vi "PrepSweepCurr.vi"(4 "OC protection":bool, 5 "Voltage/Current Limit (0V/A)":dbl, 6 "OV protection":bool, 7 "OV Value (10V)":dbl=10.0, 8 "error in (no error)":errorcluster, 9 "CC (1)/VC (0)":bool, 10 "Start Current/Voltage (0 A/V)":dbl, 11 "VISA resource name":refnum<visa-resource-name>) -> (0 "error out":errorcluster, 3 "VISA resource name out":refnum<visa-resource-name>)   [LabVIEW 2017]
doc: "Configures the current transient mode and output current level."
uses:
  Keysight N8731A conversion/Keysight N8900 Series.lvlib
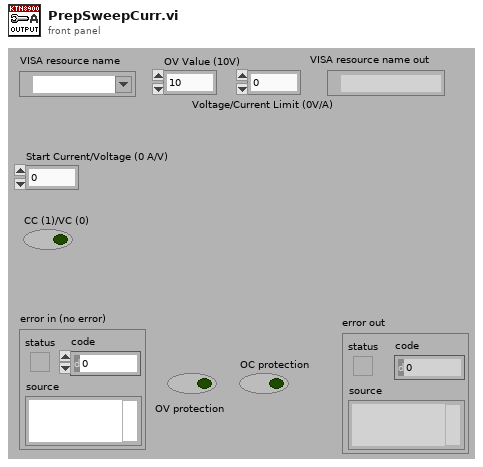
[diagram p1: front panel]
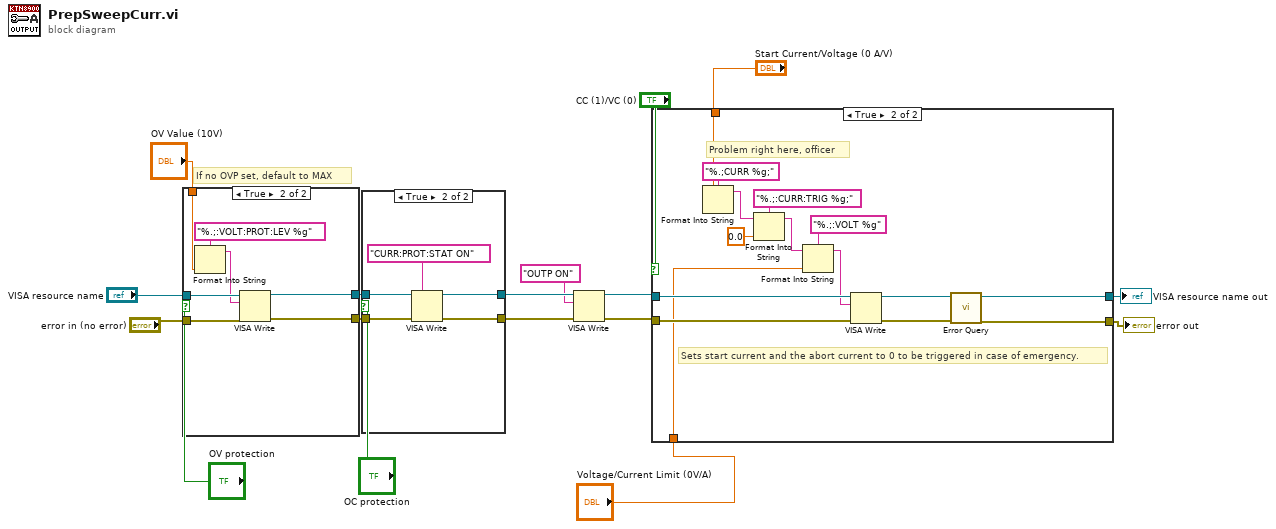
[diagram p0: block diagram]
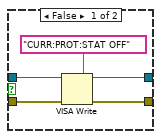
[diagram p2: hidden frame]
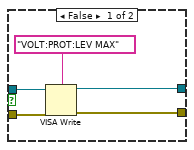
[diagram p3: hidden frame]
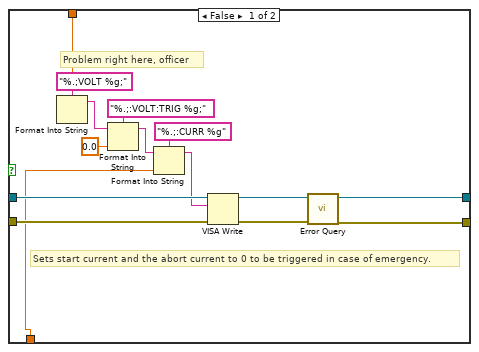
[diagram p4: hidden frame]
diagram:
  # "If no OVP set, default to MAX"
  n1 = case shown="True" "OV protection" {
    tunnel: "VISA resource name" -> [w22 w29]
    tunnel: "error in (no error)" -> [w21 w28]
    tunnel: [w19 w27] -> w13
    tunnel: [w20 w26] -> w12
    tunnel: "OV Value (10V)" -> [_ w23]
    frame False {
      n2 = VISA Write(VISA resource name=w22, write buffer="VOLT:PROT:LEV MAX", error in (no error)=w21) -> (VISA resource name out=w19:refnum<visa-resource-name>, error out=w20:errorcluster)  [unwired: 1 out]
    }
    frame True {
      n3 = Format Into String(format string="%.;:VOLT:PROT:LEV %g", w23) -> (resulting string=w24:string)  [unwired: 2 in, 1 out]
      n4 = VISA Write(VISA resource name=w29, write buffer=w24, error in (no error)=w28) -> (VISA resource name out=w27:refnum<visa-resource-name>, error out=w26:errorcluster)  [unwired: 1 out]
    }
  }
  n5 = case shown="True" "OC protection" {
    tunnel: w13 -> [w33 w39]
    tunnel: w12 -> [w32 w38]
    tunnel: [w31 w37] -> w5
    tunnel: [w30 w36] -> w4
    frame False {
      n6 = VISA Write(VISA resource name=w33, write buffer="CURR:PROT:STAT OFF", error in (no error)=w32) -> (VISA resource name out=w31:refnum<visa-resource-name>, error out=w30:errorcluster)  [unwired: 1 out]
    }
    frame True {
      n7 = VISA Write(VISA resource name=w39, write buffer="CURR:PROT:STAT ON", error in (no error)=w38) -> (VISA resource name out=w37:refnum<visa-resource-name>, error out=w36:errorcluster)  [unwired: 1 out]
    }
  }
  n8 = VISA Write(VISA resource name=w5, write buffer="OUTP ON", error in (no error)=w4) -> (VISA resource name out=w3:refnum<visa-resource-name>, error out=w2:errorcluster)  [unwired: 1 out]
  n9 = case shown="True" "CC (1)/VC (0)" {
    tunnel: w3 -> [w54 w69]
    tunnel: w2 -> [w53 w68]
    tunnel: [w50 w65] -> w9
    tunnel: [w49 w64] -> w8
    tunnel: "Start Current/Voltage (0 A/V)" -> [w44 w59]
    tunnel: "Voltage/Current Limit (0V/A)" -> [w42 w57]
    frame False {
      # "Problem right here, officer"
      # "Sets start current and the abort current to 0 to be triggered in case of emergency."
      n10 = Format Into String(format string="%.;VOLT %g;", w44) -> (resulting string=w46:string)  [unwired: 2 in, 1 out]
      n11 = Format Into String(format string="%.;:VOLT:TRIG %g;", initial string=w46, 0.0 ("input 1")) -> (resulting string=w43:string)  [unwired: 1 in, 1 out]
      n12 = Format Into String(format string="%.;:CURR %g", initial string=w43, w42) -> (resulting string=w40:string)  [unwired: 1 in, 1 out]
      n13 = VISA Write(VISA resource name=w54, write buffer=w40, error in (no error)=w53) -> (VISA resource name out=w52:refnum<visa-resource-name>, error out=w51:errorcluster)  [unwired: 1 out]
      n14 = call "Error Query.vi"("error in (no error)"=w51, "VISA resource name"=w52) -> ("error out"=w49:errorcluster, "VISA resource name out"=w50:refnum<visa-resource-name>)  [unwired: 6 in, 2 out]
    }
    frame True {
      # "Problem right here, officer"
      # "Sets start current and the abort current to 0 to be triggered in case of emergency."
      n15 = Format Into String(format string="%.;CURR %g;", w59) -> (resulting string=w61:string)  [unwired: 2 in, 1 out]
      n16 = Format Into String(format string="%.;:CURR:TRIG %g;", initial string=w61, 0.0 ("input 1")) -> (resulting string=w58:string)  [unwired: 1 in, 1 out]
      n17 = Format Into String(format string="%.;:VOLT %g", initial string=w58, w57) -> (resulting string=w56:string)  [unwired: 1 in, 1 out]
      n18 = VISA Write(VISA resource name=w69, write buffer=w56, error in (no error)=w68) -> (VISA resource name out=w67:refnum<visa-resource-name>, error out=w66:errorcluster)  [unwired: 1 out]
      n19 = call "Error Query.vi"("error in (no error)"=w66, "VISA resource name"=w67) -> ("error out"=w64:errorcluster, "VISA resource name out"=w65:refnum<visa-resource-name>)  [unwired: 6 in, 2 out]
    }
  }
  "VISA resource name out" <- w9
  "error out" <- w8
